vi "L4.vi"() -> ()   [LabVIEW 2020]
uses:
  <vilib>/vision/NI_Vision_Development_Module.lvlib
panel:
  out "Imagen FFT suma":T1(plugin-control)
  in  "Tipo FFT imagen suma":T2=3 items=["Grayscale (U8)", "Grayscale (I16)", "Grayscale (SGL)", "Complex (CSG)", "RGB (U32)", "HSL (U32)", "RGB (U64)", "Grayscale (U16)"]
  in  "Path imagen suma filtrada":path=path "C:/Users/tds013/Desktop/L4/imagen_suma_filtrada_paso_bajo.jpg"
  in  "Kernel - LPF - Boxcar":sgl[][](array[numeric])=[[1.0, 1.0, 1.0], [1.0, 1.0, 1.0], [1.0, 1.0, 1.0]] format="%.2f"
  in  "Tipo imagen filtrada":T2 items=["Grayscale (U8)", "Grayscale (I16)", "Grayscale (SGL)", "Complex (CSG)", "RGB (U32)", "HSL (U32)", "RGB (U64)", "Grayscale (U16)"]
  out "Imagen suma":T1(plugin-control)
  out "Imagen2":T1(plugin-control)
  out "Imagen1":T1(plugin-control)
  in  "Tipo imagen suma":T2 items=["Grayscale (U8)", "Grayscale (I16)", "Grayscale (SGL)", "Complex (CSG)", "RGB (U32)", "HSL (U32)", "RGB (U64)", "Grayscale (U16)"]
  in  "Tipo imagen2":T2 items=["Grayscale (U8)", "Grayscale (I16)", "Grayscale (SGL)", "Complex (CSG)", "RGB (U32)", "HSL (U32)", "RGB (U64)", "Grayscale (U16)"]
  in  "Tipo imagen1":T2 items=["Grayscale (U8)", "Grayscale (I16)", "Grayscale (SGL)", "Complex (CSG)", "RGB (U32)", "HSL (U32)", "RGB (U64)", "Grayscale (U16)"]
  in  "Path imagen 2":path=path "C:/Users/tds013/Desktop/L4/lenna_mono.tif"
  in  "Path imagen 1":path=path "C:/Users/tds013/Desktop/L4/cameraman_mono.tif"
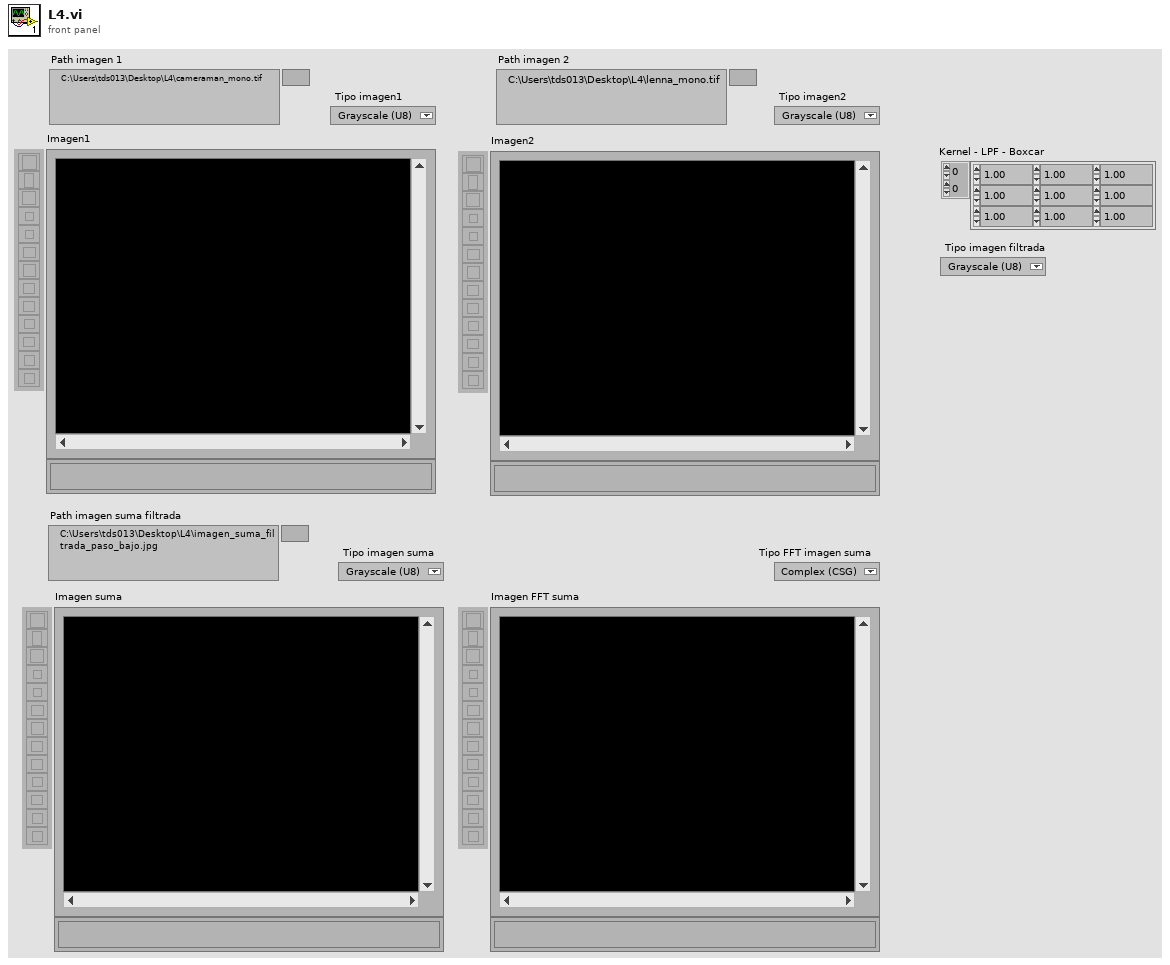
[diagram p1: front panel]
types:
  T1 = typedef "IMAQ Image.ctl" = refnum<image>
  T2 = typedef "Image Type" = u32
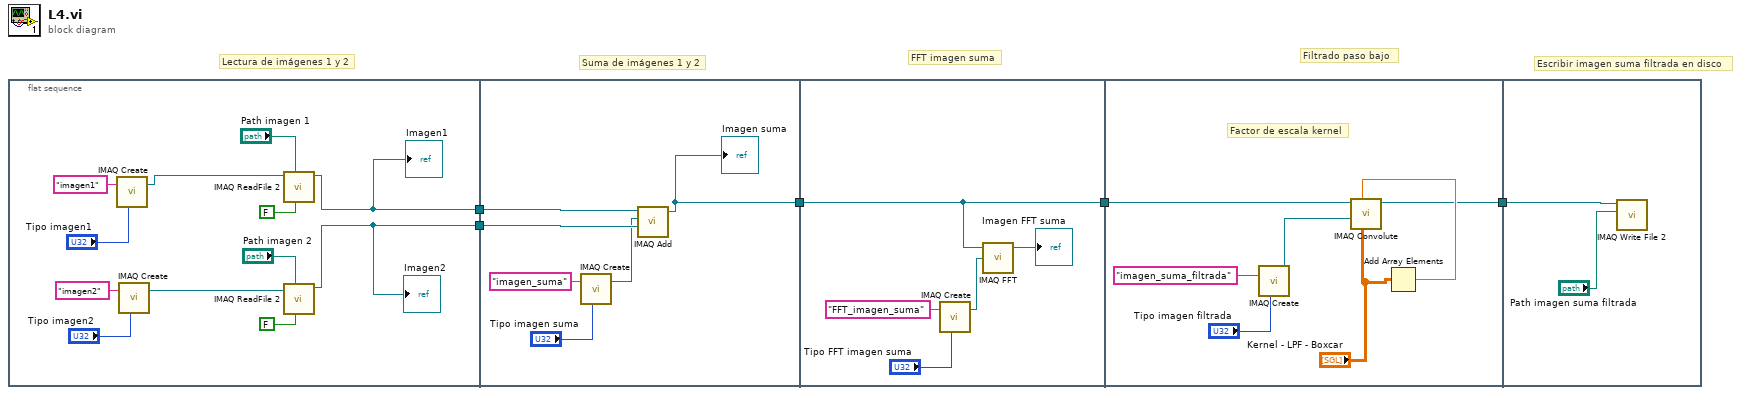
[diagram p0: block diagram]
diagram:
  # "FFT imagen suma"
  # "Escribir imagen suma filtrada en disco"
  # "Filtrado paso bajo"
  # "Suma de imágenes 1 y 2"
  # "Lectura de imágenes 1 y 2"
  n1 = flat-sequence {
    tunnel: [w7] -> w5
    tunnel: [w6] -> w4
    tunnel: w5 -> [w23]
    tunnel: w4 -> [w22]
    tunnel: [w18] -> w2
    tunnel: w2 -> [w25]
    tunnel: [w25] -> w1
    tunnel: w1 -> [w35]
    tunnel: [w29] -> w3
    tunnel: w3 -> [w37]
    frame #0 {
      n2 = call "IMAQ Create"("Image Name"="imagen1", "Image Type"="Tipo imagen1") -> ("New Image"=w12:T1)  [unwired: 3 in, 1 out]
      n3 = call "IMAQ Create"("Image Name"="imagen2", "Image Type"="Tipo imagen2") -> ("New Image"=w13:T1)  [unwired: 3 in, 1 out]
      n4 = call "IMAQ ReadFile 2"("Use File Path Image Type"=FALSE, "File Path"="Path imagen 1", "Image"=w12) -> ("Image Out"=w7:T1)  [unwired: 4 in, 4 out]
      "Imagen1" <- w7
      n5 = call "IMAQ ReadFile 2"("Use File Path Image Type"=FALSE, "File Path"="Path imagen 2", "Image"=w13) -> ("Image Out"=w6:T1)  [unwired: 4 in, 4 out]
      "Imagen2" <- w6
    }
    frame #1 {
      n6 = call "IMAQ Create"("Image Name"="imagen_suma", "Image Type"="Tipo imagen suma") -> ("New Image"=w19:T1)  [unwired: 3 in, 1 out]
      n7 = call "IMAQ Add"("Image Src A"=w23, "Image Dst"=w19, "Image Src B"=w22) -> ("Image Dst Out"=w18:T1)  [unwired: 4 in, 1 out]
      "Imagen suma" <- w18
    }
    frame #2 {
      n8 = call "IMAQ Create"("Image Name"="FFT_imagen_suma", "Image Type"="Tipo FFT imagen suma") -> ("New Image"=w26:T1)  [unwired: 3 in, 1 out]
      n9 = call "IMAQ FFT"("Image Dst"=w26, "Image Src"=w25) -> ("Image Dst Out"=→"Imagen FFT suma":T1)  [unwired: 2 in, 1 out]
    }
    frame #3 {
      # "Factor de escala kernel"
      n10 = call "IMAQ Create"("Image Name"="imagen_suma_filtrada", "Image Type"="Tipo imagen filtrada") -> ("New Image"=w32:T1)  [unwired: 3 in, 1 out]
      n11 = Add Array Elements(numeric array="Kernel - LPF - Boxcar") -> (sum=w30:sgl)
      n12 = call "IMAQ Convolute"("Kernel"="Kernel - LPF - Boxcar", "Divider (kernel sum)"=w30, "Image Dst"=w32, "Image Src"=w35) -> ("Image Dst Out"=w29:T1)  [unwired: 6 in, 1 out]
    }
    frame #4 {
      n13 = call-poly "IMAQ Write File 2"("File Path"="Path imagen suma filtrada", "Image"=w37) -> ()  [unwired: 8 in, 2 out]
    }
  }
